vi "#29_MAV_MSG_SCALED_PRESSURE_DECODE.vi"(11 "mavlink_payload":u8[](array[numeric])) -> (3 "SCALED_PRESSURE":T1)   [LabVIEW 2023]
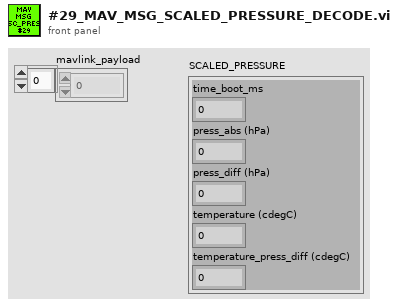
[diagram p1: front panel]
types:
  T1 = cluster{"time_boot_ms":u32, "press_abs (hPa)":sgl, "press_diff (hPa)":sgl, "temperature (cdegC)":i16, "temperature_press_diff (cdegC)":i16}
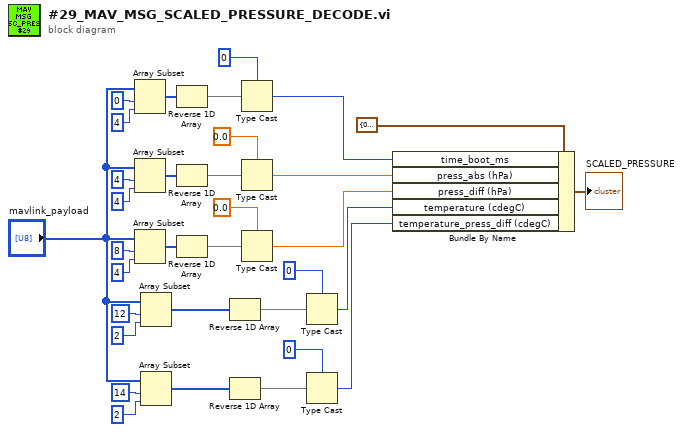
[diagram p0: block diagram]
diagram:
  n1 = Array Subset(array="mavlink_payload", index=0, length=4) -> (w31:u8[])
  n2 = Array Subset(array="mavlink_payload", index=4, length=4) -> (w23:u8[])
  n3 = Array Subset(array="mavlink_payload", index=8, length=4) -> (w17:u8[])
  n4 = Array Subset(array="mavlink_payload", index=12, length=2) -> (w11:u8[])
  n5 = Array Subset(array="mavlink_payload", index=14, length=2) -> (w5:u8[])
  n6 = Reverse 1D Array(array=w31) -> (reversed array=w30:u8[])
  n7 = Reverse 1D Array(array=w23) -> (reversed array=w22:u8[])
  n8 = Reverse 1D Array(array=w17) -> (reversed array=w16:u8[])
  n9 = Reverse 1D Array(array=w11) -> (reversed array=w10:u8[])
  n10 = Reverse 1D Array(array=w5) -> (reversed array=w4:u8[])
  n11 = Type Cast(type=u32 0 ("index"), x=w30) -> (*(type *) &x=w26:u32)
  n12 = Type Cast(type=sgl 0.0 ("index"), x=w22) -> (*(type *) &x=w20:sgl)
  n13 = Type Cast(type=sgl 0.0 ("index"), x=w16) -> (*(type *) &x=w14:sgl)
  n14 = Type Cast(type=i16 0 ("index"), x=w10) -> (*(type *) &x=w8:i16)
  n15 = Type Cast(type=i16 0 ("index"), x=w4) -> (*(type *) &x=w1:i16)
  n16 = Bundle By Name(cluster=T1 {"time_boot_ms"=0, "press_abs (hPa)"=0.0, "press_diff (hPa)"=0.0, "temperature (cdegC)"=0, "temperature_press_diff (cdegC)"=0} ("SCALED_PRESSURE"), "time_boot_ms"=w26, "press_abs (hPa)"=w20, "press_diff (hPa)"=w14, "temperature (cdegC)"=w8, "temperature_press_diff (cdegC)"=w1) -> (→"SCALED_PRESSURE":T1)
